vi "CheckMutationHistory.vi"() -> ()   [LabVIEW 2020]
uses:
  <vilib>/Utility/EditLVLibs/Edit LVLibs.lvlib
panel:
  in  "Also Clear the history(False)":bool
  out "Classes":cluster{"Numeric":i32, "name":string}[](array[cluster])
  # "No Of Mut History"
  # "Class name"
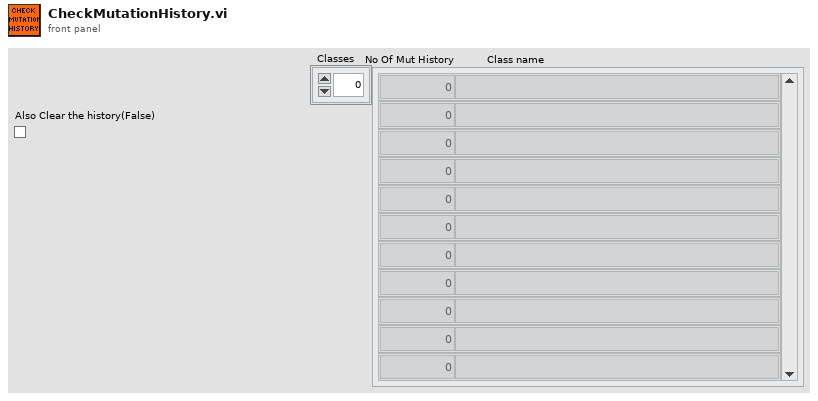
[diagram p1: front panel]
types:
  T1 = typedef "Edit LVLibs.lvlib/Mutation History.ctl" = T2[]
  T2 = typedef "Edit LVLibs.lvlib/Mutation Record.ctl" = cluster{"Library Version":T3, "Old Name Index":u8, "Class Default Data":variant, "Cluster Order Map":u32[], "Parent Name":string, "Parent Path":path, "LabVIEW Version":u32, "User Comments":string, "Mutation Flags":u8, "Parent Old Name Index":u8, "Parent Levels Added":u16, "Parent Levels Removed":u16}
  T3 = typedef "Edit LVLibs.lvlib/LibVersion.ctl" = cluster{"Major":u16, "Minor":u16, "Fix":u16, "Build":u16}
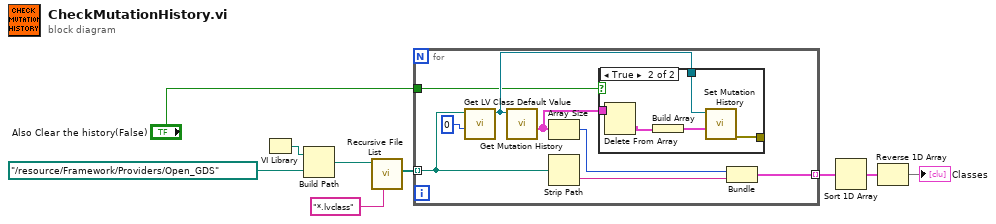
[diagram p0: block diagram]
diagram:
  n1 = VI Library() -> (path=w9:path)
  n2 = Build Path(base path=w9, name or relative path=path "../resource/Framework/Providers/Open_GDS") -> (appended path=w4:path)
  n3 = call <vilib>:"Recursive File List.vi"("pattern"="*.lvclass", "Folder Path"=w4) -> ("All Files in Dir"=w2:path[])  [unwired: 5 in, 4 out]
  n4 = for {
    tunnel: [w14] -> w7 mode=indexing
    tunnel: w2 -> [w13] mode=indexing
    tunnel: "Also Clear the history(False)" -> [w10]
    n5 = call <vilib>:"Get LV Class Default Value.vi"("options"=u32 0, "class path"=w13) -> ("object"=w11:refnum<class>)  [unwired: 8 in, 1 out]
    n6 = call <vilib>:"Get Mutation History.vi"("Input object"=w11) -> ("Mutation History"=w12:T1)  [unwired: 7 in, 1 out]
    n7 = Array Size(array=w12) -> (size(s)=w16:i32)
    n8 = Strip Path(path=w13) -> (name=w15:string)  [unwired: 1 out]
    n9 = case shown="True" w10 {
      tunnel: w12 -> [_ w21]
      tunnel: w11 -> [_ w19]
      tunnel: [_ w18] -> _
      frame False {
      }
      frame True {
        n10 = Delete From Array(array=w21) -> (deleted portion=w20:T2)  [unwired: 2 in, 1 out]
        n11 = Build Array(w20) -> (w22:T2[])
        n12 = call <vilib>:"Set Mutation History.vi"("Mutation History"=w22, "Input object"=w19) -> ("error out"=w18:errorcluster)  [unwired: 9 in]
      }
    }
    n13 = Bundle(w16, "name"=w15) -> (w14:cluster{i32, "name":string})  [unwired: 1 in]
  }
  n14 = Sort 1D Array(array=w7) -> (sorted array=w6:cluster{i32, "name":string}[])
  n15 = Reverse 1D Array(array=w6) -> (reversed array=→"Classes":cluster{i32, "name":string}[])
